vi "SaveFile.vi"(9 "stop":bool, 10 "Numeric":dbl, 11 "Path":path) -> (0 "error out":errorcluster, 1 "data":string)   [LabVIEW 2019]
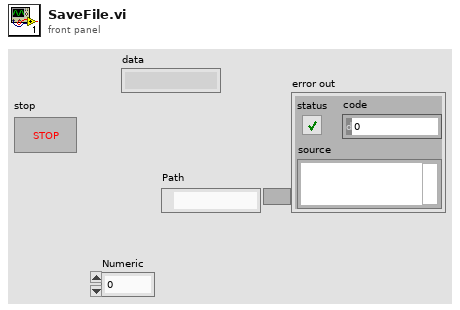
[diagram p1: front panel]
types:
  T1 = enum16{"open", "replace", "create", "open or create", "replace or create", "replace or create with confirmation"}
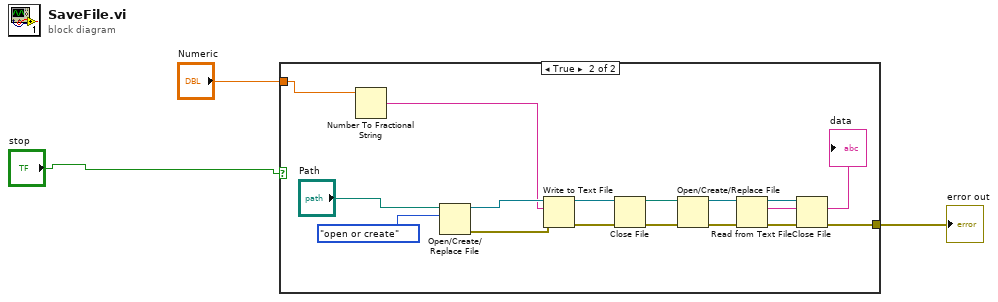
[diagram p0: block diagram]
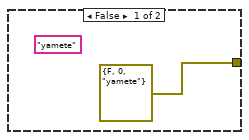
[diagram p2: hidden frame]
diagram:
  n1 = case shown="True" "stop" {
    tunnel: "Numeric" -> [_ w6]
    tunnel: [errorcluster {"status"=FALSE, "code"=0, "source"="yamete"} ("error out") w8] -> w2
    frame False {
      (unwired) "yamete"
    }
    frame True {
      n2 = Number To Fractional String(number=w6) -> (F-format string=w5:string)  [unwired: 3 in]
      n3 = Open/Create/Replace File(file path (use dialog)="Path", operation (0:open)=T1."open or create") -> (refnum out=w19:refnum<file>, error out=w13:errorcluster)  [unwired: 4 in, 1 out]
      n4 = Write to Text File(file (use dialog)=w19, text=w5, error in=w13) -> (refnum out=w20:refnum<file>, error out=w12:errorcluster)  [unwired: 1 in, 1 out]
      n5 = Close File(refnum=w20, error in=w12) -> (path=w16:path, error out=w11:errorcluster)
      n6 = Open/Create/Replace File(file path (use dialog)=w16, error in=w11) -> (refnum out=w15:refnum<file>, error out=w10:errorcluster)  [unwired: 4 in, 1 out]
      n7 = Read from Text File(file (use dialog)=w15, error in=w10) -> (refnum out=w17:refnum<file>, text=→"data":string, error out=w9:errorcluster)  [unwired: 2 in, 1 out]
      n8 = Close File(refnum=w17, error in=w9) -> (error out=w8:errorcluster)  [unwired: 1 out]
    }
  }
  "error out" <- w2
